vi "Slave - Interleaved Chs Throughput.vi"() -> ()   [LabVIEW 2016]
uses:
  <vilib>/Utility/error.llb/DialogType.ctl
  <vilib>/pximc/Initialize Writer Session (DBL).vi
  <vilib>/pximc/Connect (DBL).vi
  <vilib>/pximc/Acquire Write Region (DBL).vi
  <vilib>/pximc/nipximc.lvlib
panel:
  out "Throughput S/s":dbl format="%#.2p"
  out "Time has Elapsed":bool
  in  "Stop Button":bool
  in  "#Writing Channels Slave 1":i32=2
  in  "Node 1 Writer Connection ID":u16=1
  in  "Node 1 Writer Interface":tag="PXIMC2" caption="interface"
  in  "Connection Timeout (s)":dbl=60.0 caption="timeout in seconds (-1)"
  # "Node 1"
  # "Node 2 => Node 1"
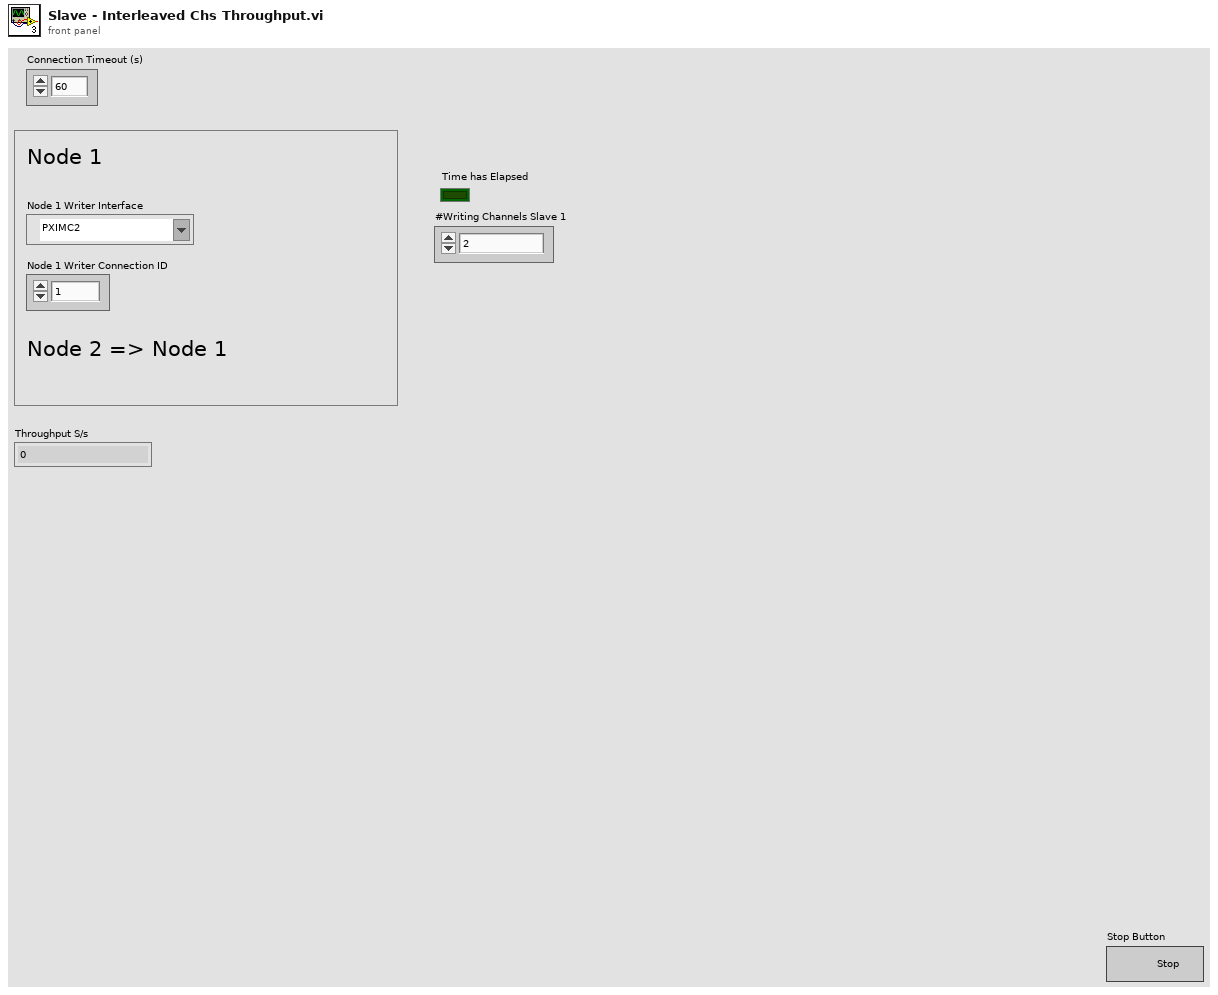
[diagram p1: front panel]
types:
  T1 = typedef "DialogType.ctl" = u16
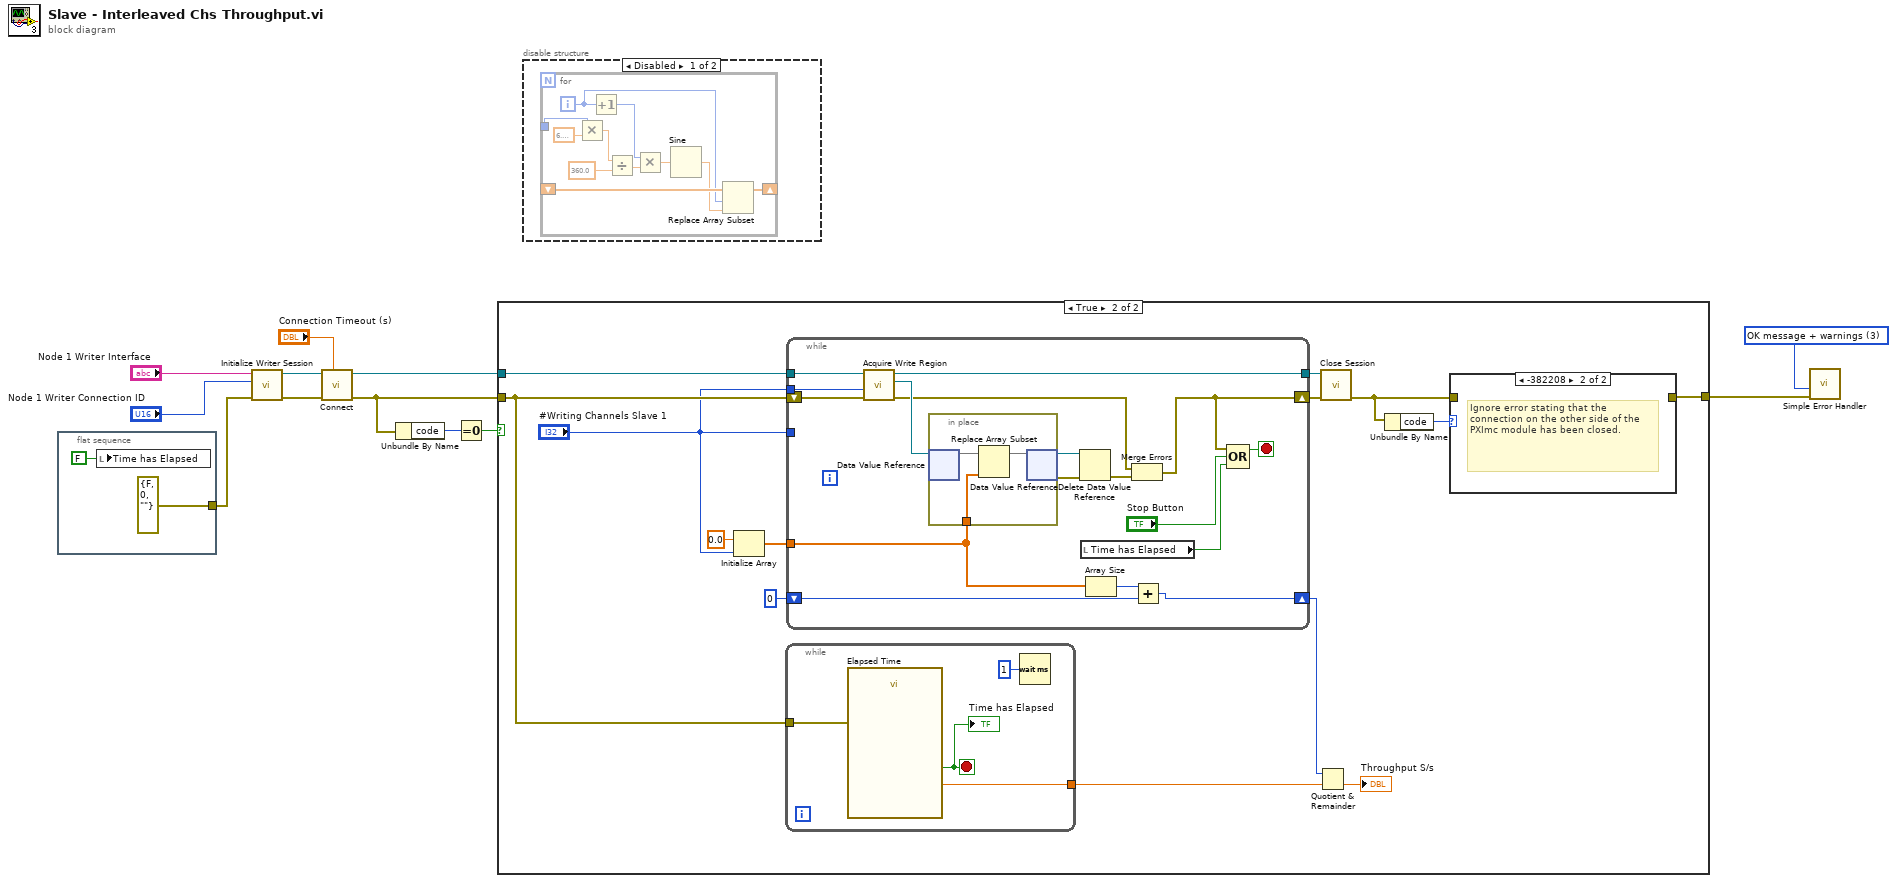
[diagram p0: block diagram]
diagram:
  w12 = T1 3 items=["no dialog", "OK message", "continue or stop message", "OK message + warnings", "continue/stop + warnings"] ("type of dialog (OK msg:1)")
  n1 = flat-sequence {
    tunnel: [errorcluster {"status"=FALSE, "code"=0, "source"=""} ("error constant")] -> w5
    frame #0 {
      n2 = local write "Time has Elapsed"(FALSE ("Stopped?")) -> ()
    }
  }
  n3 = call-poly <vilib>:"Initialize Writer Session.vi"("error in (no error)"=w5, "connection id (1)"="Node 1 Writer Connection ID", "interface"="Node 1 Writer Interface") -> ("error out"=w10:errorcluster, "session out"=w9:refnum<k21>)  [unwired: 7 in]
  n4 = call-poly <vilib>:"Connect.vi"("timeout in seconds (-1)"="Connection Timeout (s)", "error in (no error)"=w10, "session in"=w9) -> ("error out"=w1:errorcluster, "session out"=w6:refnum<k21>)  [unwired: 7 in]
  n5 = Unbundle By Name(w1) -> ("code"=w7:i32)
  n6 = Equal To 0?(x=w7) -> (x = 0?=w2:bool)
  n7 = case shown="True" w2 {
    tunnel: [w15 w29] -> w4
    tunnel: w6 -> [_ w27]
    tunnel: w1 -> [w15 w22]
    frame False {
      # "The connection was not successful for some reason."
    }
    frame True {
      n8 = Initialize Array(0.0 ("element"), "#Writing Channels Slave 1") -> (w17:dbl[])
      n9 = while {
        tunnel: w22 -> [w32]
        tunnel: [w31] -> w20
        stop <- w33 stop-if-true
        n10 = call "Elapsed Time"("error in (no error)"=w32) -> ("Elapsed Time (s)"=w31:dbl, "Time has Elapsed"=w33:bool)  [unwired: 11 in, 6 out]
        "Time has Elapsed" <- w33
        n11 = Wait (ms)(milliseconds to wait=u32 1) -> ()  [unwired: 1 out]
      }
      n12 = while {
        tunnel: w27 -> [w45]
        tunnel: [w44] -> w26
        shift-right: [w42] -> w25
        shift-left: w22 -> [w43]
        shift-right: [w38] -> w21
        shift-left: u32 0 ("element") -> [w39]
        tunnel: w17 -> [w34]
        tunnel: "#Writing Channels Slave 1" -> [w35]
        tunnel: "#Writing Channels Slave 1" -> [_]
        stop <- w41 stop-if-true
        n13 = call-poly <vilib>:"Acquire Write Region.vi"("error in (no error)"=w43, "number of elements"=w35, "session in"=w45) -> ("error out"=w46:errorcluster, "write region reference"=w47:refnum<data-value>, "session out"=w44:refnum<k21>)  [unwired: 5 in, 1 out]
        n14 = in-place {
          in-place-border: w34 -> [w51]
          n15 = in-place-dvr #1(w47) -> (w53:dbl[])  [unwired: 1 out]
          n16 = Replace Array Subset(array=w53, new element=w51) -> (w52:dbl[])  [unwired: 1 in]
          n17 = in-place-dvr #1(w52) -> (w48:refnum<data-value>, w50:errorcluster)
        }
        n18 = Delete Data Value Reference(data value reference=w48, error in=w50) -> (error out=w49:errorcluster)  [unwired: 1 out]
        n19 = local read "Time has Elapsed"() -> (w37:bool)
        n20 = Array Size(array=w34) -> (size(s)=w36:i32)
        n21 = Merge Errors(w46, w49) -> (w42:errorcluster)
        n22 = Add(x=w36, y=w39) -> (x+y=w38:u32)
        n23 = Compound Arithmetic op=OR(w42, "Stop Button", w37) -> (w41:bool)
      }
      n24 = Quotient & Remainder(x=w21, y=w20) -> (floor(x/y)=→"Throughput S/s":dbl)  [unwired: 1 out]
      n25 = call <vilib>:"Close Session.vi"("error in (no error)"=w25, "session in"=w26) -> ("error out"=w24:errorcluster)  [unwired: 9 in]
      n26 = Unbundle By Name(w24) -> ("code"=w28:i32)
      n27 = case shown="-382208" w28 {
        tunnel: w24 -> [w54 _]
        tunnel: [w54 _] -> w29
        frame 0, Default {
        }
        frame -382208 {
          # "Ignore error stating that the connection on the other side of the PXImc module has been closed."
        }
      }
    }
  }
  n28 = disable-structure shown="Disabled" {
    frame Disabled {
      n29 = for {
        tunnel: _ -> [w59]
        shift-right: [w57] -> _
        shift-left: _ -> [w58]
        i -> [w55]
        n30 = Multiply(x=w59, y=6.283185307179586) -> (x*y=w62:dbl)
        n31 = Increment(x=w55) -> (x+1=w60:i32)
        n32 = Divide(x=w62, y=360.0) -> (x/y=w64:dbl)
        n33 = Multiply(x=w60, y=w64) -> (x*y=w65:dbl)
        n34 = Sine(x=w65) -> (sin(x)=w56:dbl)
        n35 = Replace Array Subset(array=w58, new element=w56, index=w55) -> (w57:dbl[])
      }
    }
    frame Enabled {
    }
  }
  n36 = call <vilib>:"Simple Error Handler.vi"("type of dialog (OK msg:1)"=w12, "error in (no error)"=w4) -> ()  [unwired: 3 in, 5 out]
